vi "disk_GetTemplate.vi"(8 "error in (no error)":errorcluster, 11 "file path":path=path "C:/test.xlsx") -> (0 "error out":errorcluster, 3 "DiskTemplate":T1)   [LabVIEW 2017, in "NI_ExcelFile.lvlib"]
uses:
  <vilib>/express/express shared/NI_ExcelFile/NI_ExcelFile.lvlib
  <vilib>/express/express shared/NI_ExcelFile/Ctrls/disk_TemplateFile.ctl
  <vilib>/express/express shared/NI_ExcelFile/Ctrls/meta_file.ctl
  <vilib>/express/express shared/NI_ExcelFile/Ctrls/meta_Block.ctl
  <vilib>/express/express shared/NI_ExcelFile/Ctrls/meta_BlockType.ctl
  <vilib>/express/express shared/NI_ExcelFile/Ctrls/TemplateEnum.ctl
  <vilib>/zip/NI_Unzip.lvlib
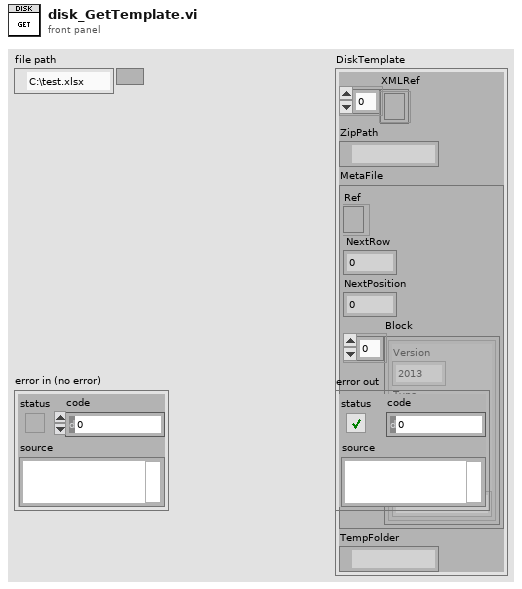
[diagram p1: front panel]
types:
  T1 = typedef "NI_ExcelFile.lvlib/disk_TemplateFile.ctl" = cluster{"XMLRef":refnum<file>[], "ZipPath":path, "MetaFile":T2, "TempFolder":path}
  T2 = typedef "NI_ExcelFile.lvlib/meta_file.ctl" = cluster{"Ref":refnum<file>, "NextRow":i32, "NextPosition":i64, "Block":T3[]}
  T3 = typedef "NI_ExcelFile.lvlib/meta_Block.ctl" = cluster{"Version":u16, "Type":T4, "Length":i32, "Data":string}
  T4 = typedef "NI_ExcelFile.lvlib/meta_BlockType.ctl" = enum16{"NITag", "File", "Column"}
  T5 = typedef "NI_ExcelFile.lvlib/TemplateEnum.ctl" = enum16{"[Content_Types].xml", ".rels", "workbook.xml", "styles.xml", "workbook.xml.rels", "sheet.xml", "app.xml", "core.xml"}
  T6 = typedef "NI_ExcelFile.lvlib/meta_FileInfo.ctl" = cluster{"meta_FileInfo_2013":T7}
  T7 = typedef "NI_ExcelFile.lvlib/meta_FileInfo_2013.ctl" = cluster{"NextPosition":i64, "NextRow":i32, "FileAttribute ":T8}
  T8 = typedef "NI_ExcelFile.lvlib/FileAttribute.ctl" = cluster{"Creator":string, "Title":string, "SheetName":string}
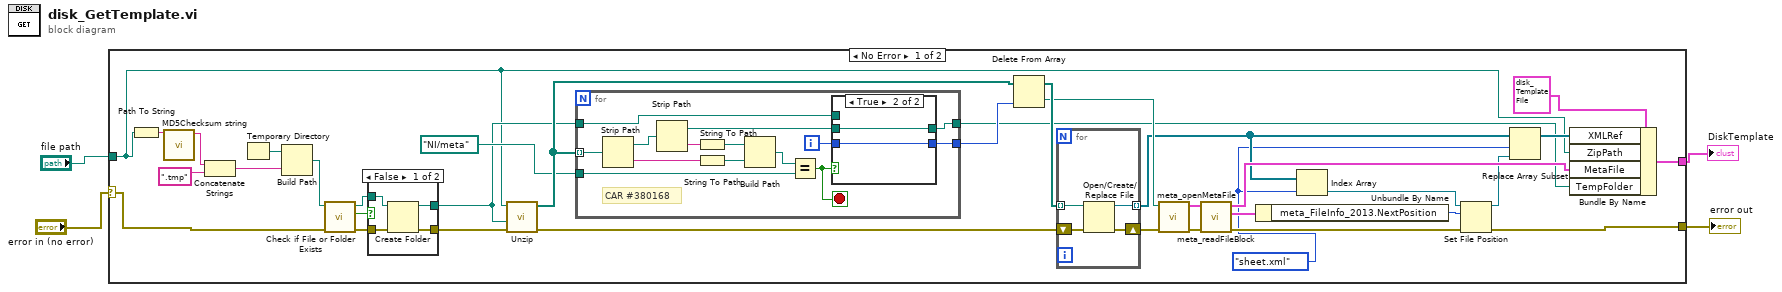
[diagram p0: block diagram]
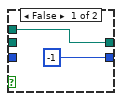
[diagram p2: hidden frame]
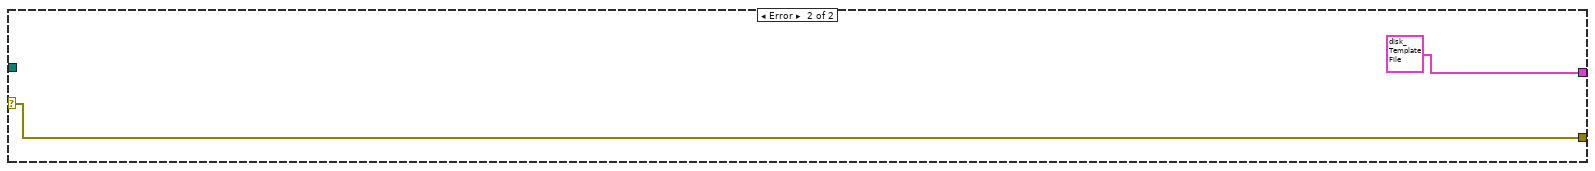
[diagram p4: hidden frame]
diagram:
  n1 = case shown="No Error" "error in (no error)" {
    selector: "error in (no error)" -> [w14 w69]
    tunnel: [w36 T1 {"XMLRef"=[refnum, refnum, refnum, refnum, refnum, refnum], "ZipPath"=path "", "MetaFile"={"Ref"=refnum, "NextRow"=0, "NextPosition"=0, "Block"=[]}, "TempFolder"=path ""} ("XLSX file")] -> w4
    tunnel: "file path" -> [w6 _]
    tunnel: [w19 w69] -> w2
    frame No Error {
      w13 = TemplateEnum."sheet.xml" ("Template")
      n2 = Path To String(path=w6) -> (string=w7:string)
      n3 = call <vilib>:"MD5Checksum string.vi"("Message String"=w7) -> ("MD5 message-digest"=w5:string)  [unwired: 10 in]
      n4 = Concatenate Strings(w5, ".tmp" ("string")) -> (w32:string)
      n5 = Temporary Directory() -> (w31:path)
      n6 = Build Path(base path=w31, name or relative path=w32) -> (appended path=w29:path)
      n7 = call <vilib>:"Check if File or Folder Exists.vi"("error in (no error)"=w14, "path"=w29) -> ("error out"=w26:errorcluster, "file or folder exists?"=w28:bool, "dup path"=w27:path)  [unwired: 7 in]
      n8 = case shown="False" w28 {
        tunnel: w27 -> [w61 w63]
        tunnel: w26 -> [w60 w62]
        tunnel: [w59 w62] -> w25
        tunnel: [w58 w63] -> w9
        frame False {
          n9 = Create Folder(path (use dialog)=w61, error in=w60) -> (created path=w58:path, error out=w59:errorcluster)  [unwired: 1 in, 1 out]
        }
        frame True {
        }
      }
      n10 = call <vilib>:"Unzip.vi"("error in (no error)"=w25, "Target directory (same as Zip file if empty)"=w9, "Zip file"=w6) -> ("error out"=w39:errorcluster, "Unzipped files"=w12:path[])  [unwired: 6 in, 1 out]
      n11 = for {
        tunnel: w12 -> [w48] mode=indexing
        tunnel: path "NI/meta" ("element") -> [w46]
        tunnel: [w43] -> w10
        tunnel: w9 -> [w42]
        tunnel: [w40] -> w8
        i -> [w44]
        stop <- w45 stop-if-true
        # "CAR #380168"
        n12 = Strip Path(path=w48) -> (stripped path=w53:path, name=w52:string)
        n13 = Strip Path(path=w53) -> (stripped path=w41:path, name=w51:string)
        n14 = String To Path(string=w51) -> (path=w50:path)
        n15 = String To Path(string=w52) -> (path=w49:path)
        n16 = Build Path(base path=w50, name or relative path=w49) -> (appended path=w47:path)
        n17 = Equal?(x=w47, y=w46) -> (x = y?=w45:bool)
        n18 = case shown="True" w45 {
          tunnel: w44 -> [_ w57]
          tunnel: [-1 w57] -> w43
          tunnel: w42 -> [w54 _]
          tunnel: w41 -> [_ w56]
          tunnel: [w54 w56] -> w40
          frame False {
          }
          frame True {
          }
        }
      }
      n19 = Delete From Array(array=w12, index=w10) -> (deleted portion=w23:path, array with subset deleted=w30:path[])  [unwired: 1 in]
      n20 = for {
        tunnel: w30 -> [w64] mode=indexing
        tunnel: [w65] -> w22 mode=indexing
        shift-right: [w66] -> w37
        shift-left: w39 -> [w67]
        n21 = Open/Create/Replace File(file path (use dialog)=w64, error in=w67) -> (refnum out=w65:refnum<file>, error out=w66:errorcluster)  [unwired: 4 in, 1 out]
      }
      n22 = call <vilib>:"meta_openMetaFile.vi"("error in"=w37, "path"=w23) -> ("error out"=w34:errorcluster, "meta file"=w35:T2)  [unwired: 8 in]
      n23 = call <vilib>:"meta_readFileBlock.vi"("error in (no error)"=w34, "meta file in"=w35) -> ("error out"=w20:errorcluster, "file info"=w18:T6, "meta file out"=w24:T2)  [unwired: 7 in]
      n24 = Unbundle By Name(w18) -> ("meta_FileInfo_2013.NextPosition"=w17:i64)
      n25 = Index Array(array=w22, index=w13) -> (element=w16:refnum<file>)
      n26 = Set File Position(offset (in bytes) (0)=w17, refnum=w16, error in=w20) -> (refnum out=w15:refnum<file>, error out=w19:errorcluster)  [unwired: 1 in]
      n27 = Replace Array Subset(array=w22, new element=w15, index=w13) -> (w21:refnum<file>[])
      n28 = Bundle By Name(cluster=T1 {"XMLRef"=[refnum, refnum, refnum, refnum, refnum, refnum], "ZipPath"=path "", "MetaFile"={"Ref"=refnum, "NextRow"=0, "NextPosition"=0, "Block"=[]}, "TempFolder"=path ""} ("XLSX file"), "XMLRef"=w21, "ZipPath"=w6, "MetaFile"=w24, "TempFolder"=w8) -> (w36:T1)
    }
    frame Error {
    }
  }
  "DiskTemplate" <- w4
  "error out" <- w2
